vi "Auto Drive.vi"(9 "Speed":dbl=0.5, 10 "Amount":dbl, 11 "Run?":bool) -> (3 "Done":bool)   [LabVIEW 2013]
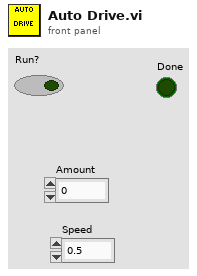
[diagram p1: front panel]
types:
  T1 = typedef "WPI_MotorControlDeviceRef.ctl" = cluster{"DeviceStatus":errorcluster, "Type":enum16{"PWM", "CAN"}, "PWM":cluster{"Digital Module":T2, "PWM Channel":T3, "DeadBand":T4}, "CAN":cluster{"Device Number":u8, "Control Mode":T5, "Semaphore":T6, "Max Vout":dbl}, "Invert":bool, "TransformRef":T7, "InvTransformRef":T7}
  T2 = typedef "FPGA_TypedefDigitalModule.ctl" = enum16{"Digital Module 1", "Digital Module 2"}
  T3 = typedef "FPGA_DIOPWMChannel.ctl" = enum8{"PWM 1", "PWM 2", "PWM 3", "PWM 4", "PWM 5", "PWM 6", "PWM 7", "PWM 8", "PWM 9", "PWM 10", "Invalid"}
  T4 = typedef "WPI_PWMDeadband.ctl" = cluster{"Name":string, "maxPositivePwm":i32, "minPositivePwm":i32, "centerPwm":i32, "maxNegativePwm":i32, "minNegativePwm":i32, "angularRange":u16}
  T5 = typedef "WPI_CANJaguar_ControlMode.ctl" = enum8{"Percent VBus", "Current", "Speed", "Position", "Voltage"}
  T6 = typedef "Semaphore RefNum" = refnum<k1>
  T7 = typedef "WPI_PWMTransform_ConPane.ctl" = refnum<vi>
  T8 = typedef "WPI_EncoderDevRef.ctl" = cluster{"DevStatus":errorcluster, "EncoderIndex":T9, "CounterIndex":T10, "DistancePerCount":dbl, "Decoding Type":T11}
  T9 = typedef "FPGA_EncoderIdx.ctl" = enum8{"Enc 0", "Enc 1", "Enc 2", "Enc 3", "Invalid"}
  T10 = typedef "FPGA_CounterCtrSystemIndex.ctl" = enum8{"Ctr 0", "Ctr 1", "Ctr 2", "Ctr 3", "Ctr 4", "Ctr 5", "Ctr 6", "Ctr 7", "Invalid"}
  T11 = typedef "WPI_EncoderType.ctl" = enum16{"1x", "2x", "4x"}
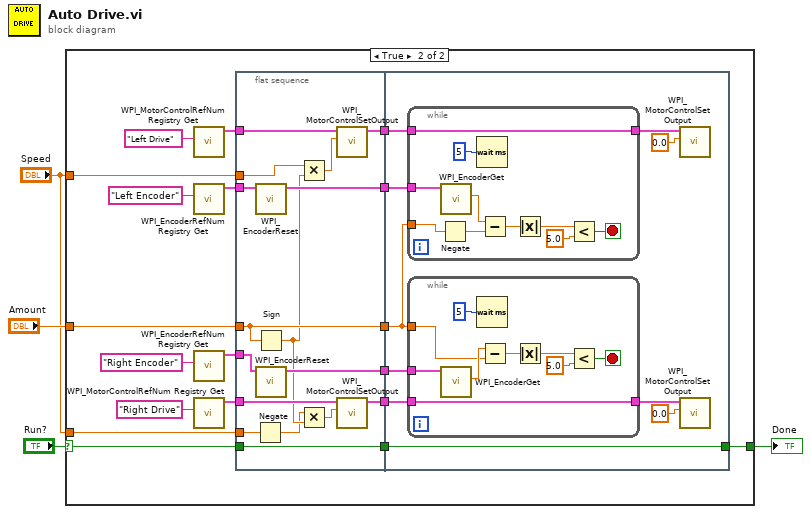
[diagram p0: block diagram]
diagram:
  n1 = case shown="True" "Run?" {
    selector: "Run?" -> [w5 w10]
    tunnel: [w5 w9] -> w3
    tunnel: "Amount" -> [_ w11]
    tunnel: "Speed" -> [_ w7]
    tunnel: "Speed" -> [_ w6]
    frame False {
    }
    frame True {
      n2 = call <vilib>:"WPI_MotorControlRefNum Registry Get.vi"("refnum name"="Left Drive") -> ("MotorControlDevRef"=w13:T1)  [unwired: 9 in, 1 out]
      n3 = call <vilib>:"WPI_EncoderRefNum Registry Get.vi"("refnum name"="Left Encoder") -> ("EncoderDevRef"=w20:T8)  [unwired: 9 in, 1 out]
      n4 = call <vilib>:"WPI_EncoderRefNum Registry Get.vi"("refnum name"="Right Encoder") -> ("EncoderDevRef"=w18:T8)  [unwired: 9 in, 1 out]
      n5 = call <vilib>:"WPI_MotorControlRefNum Registry Get.vi"("refnum name"="Right Drive") -> ("MotorControlDevRef"=w16:T1)  [unwired: 9 in, 1 out]
      n6 = flat-sequence {
        tunnel: w13 -> [w40]
        tunnel: w16 -> [w39]
        tunnel: [w38] -> w24
        tunnel: [w37] -> w23
        tunnel: [w33] -> w22
        tunnel: w18 -> [w34]
        tunnel: [w35] -> w21
        tunnel: w20 -> [w36]
        tunnel: [w31] -> w12
        tunnel: w11 -> [w31]
        tunnel: w10 -> [w32]
        tunnel: [w32] -> w8
        tunnel: w7 -> [w26]
        tunnel: w6 -> [w25]
        tunnel: w24 -> [w48]
        tunnel: w23 -> [w47]
        tunnel: w22 -> [w50]
        tunnel: w21 -> [w49]
        tunnel: w12 -> [w42]
        tunnel: [w41] -> w9
        tunnel: w8 -> [w41]
        frame #0 {
          n7 = Negate(x=w25) -> (-x=w27:dbl)
          n8 = call <vilib>:"WPI_EncoderReset.vi"("EncoderDevRef"=w36) -> ("EncoderDevRef"=w35:T8)  [unwired: 9 in, 1 out]
          n9 = Sign(1:w31) -> (0:w29:dbl)
          n10 = call <vilib>:"WPI_EncoderReset.vi"("EncoderDevRef"=w34) -> ("EncoderDevRef"=w33:T8)  [unwired: 9 in, 1 out]
          n11 = Multiply(x=w26, y=w29) -> (x*y=w28:dbl)
          n12 = Multiply(x=w27, y=w29) -> (x*y=w30:dbl)
          n13 = call <vilib>:"WPI_MotorControlSetOutput.vi"("Output"=w28, "MotorControlDevRef"=w40) -> ("MotorControlDevRef"=w38:T1)  [unwired: 7 in, 2 out]
          n14 = call <vilib>:"WPI_MotorControlSetOutput.vi"("Output"=w30, "MotorControlDevRef"=w39) -> ("MotorControlDevRef"=w37:T1)  [unwired: 7 in, 2 out]
        }
        frame #1 {
          n15 = while {
            tunnel: w49 -> [w59]
            tunnel: w48 -> [w58]
            tunnel: [w58] -> w44
            tunnel: w42 -> [w52]
            stop <- w53 stop-if-true
            n16 = Negate(x=w52) -> (-x=w51:dbl)
            n17 = call <vilib>:"WPI_EncoderGet.vi"("EncoderDevRef"=w59) -> ("Distance"=w54:dbl)  [unwired: 5 in, 5 out]
            n18 = Wait (ms)(milliseconds to wait=u32 5) -> ()  [unwired: 1 out]
            n19 = Subtract(x=w54, y=w51) -> (x-y=w56:dbl)
            n20 = Absolute Value(x=w56) -> (abs(x)=w55:dbl)
            n21 = Less?(x=w55, y=5.0) -> (x < y?=w53:bool)
          }
          n22 = while {
            tunnel: w50 -> [w68]
            tunnel: [w67] -> w46
            tunnel: w47 -> [w67]
            tunnel: w42 -> [w61]
            stop <- w62 stop-if-true
            n23 = call <vilib>:"WPI_EncoderGet.vi"("EncoderDevRef"=w68) -> ("Distance"=w66:dbl)  [unwired: 5 in, 5 out]
            n24 = Wait (ms)(milliseconds to wait=u32 5) -> ()  [unwired: 1 out]
            n25 = Subtract(x=w66, y=w61) -> (x-y=w65:dbl)
            n26 = Absolute Value(x=w65) -> (abs(x)=w64:dbl)
            n27 = Less?(x=w64, y=5.0) -> (x < y?=w62:bool)
          }
          n28 = call <vilib>:"WPI_MotorControlSetOutput.vi"("Output"=0.0, "MotorControlDevRef"=w44) -> ()  [unwired: 7 in, 3 out]
          n29 = call <vilib>:"WPI_MotorControlSetOutput.vi"("Output"=0.0, "MotorControlDevRef"=w46) -> ()  [unwired: 7 in, 3 out]
        }
      }
    }
  }
  "Done" <- w3
